vi "Register Broadcast.vi"(0 "CSM Name":string, 1 "TcpRouter-Client in":refnum<class "TcpRouter-Client.lvclass">, 5 "Source CSM Name (* as Default)":string="*", 7 "Status":string, 9 "Response Message (if \"\", same as Source Message)":string, 11 "error in (no error)":errorcluster, 12 "Response Timeout(5000ms)":i32=5000, 13 "Priority (No Change)":T1) -> (4 "CSM Name(dup)":string, 15 "error out":errorcluster)   [LabVIEW 2020, in "CSM-TCP-Router.lvlib" / "TcpRouter-Client.lvclass"]
uses:
  TcpRouter-Client.lvclass
  TcpRouter-Client.lvclass/TcpRouter-Client.ctl
  CSM-TCP-Router.lvlib
  _support/tcp-msg type.ctl
  <userlib>/_NEVSTOP/Communicable State Machine(CSM)/Communicable State Machine.lvlib
  f32241c3-0036-4787-bc41-e9c1f987f5e1.vi
  <userlib>/_NEVSTOP/Communicable State Machine(CSM)/_Polymophic/Build Register Message.vi
  <userlib>/_NEVSTOP/Communicable State Machine(CSM)/AdvanceAPI/CSM - Broadcast Message Type.ctl
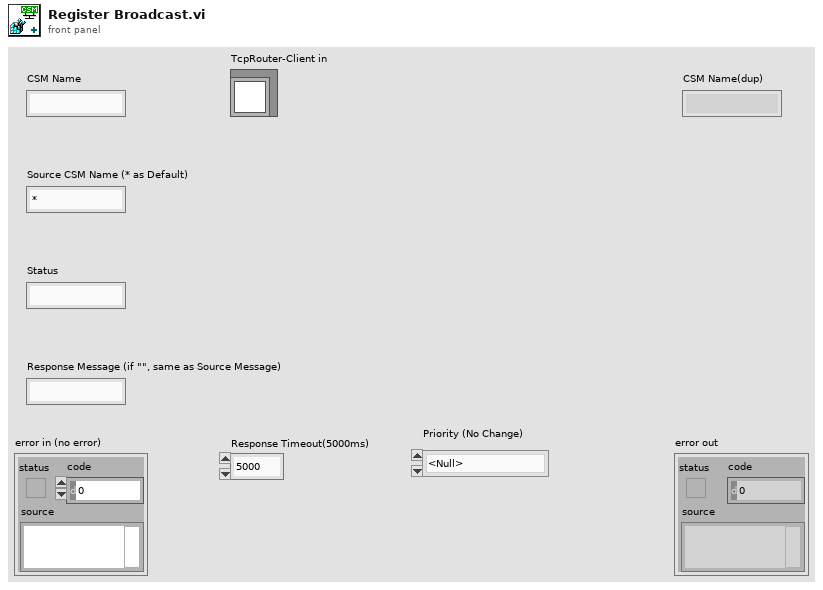
[diagram p1: front panel]
types:
  T1 = typedef "Communicable State Machine.lvlib/CSM - Broadcast Message Type.ctl" = enum16{"<Null>", "Status", "Interrupt"}
  T2 = typedef "CSM-TCP-Router.lvlib/tcp-msg type.ctl" = enum8{"info", "error", "cmd", "cmd-resp", "resp", "async-resp", "status", "interrupt"}
  T3 = typedef "CSM-TCP-Router.lvlib/TcpRouter-Client.lvclass/Def-TCP-Router REQ-REP.ctl" = cluster{"REQ-REP":refnum<k5>}
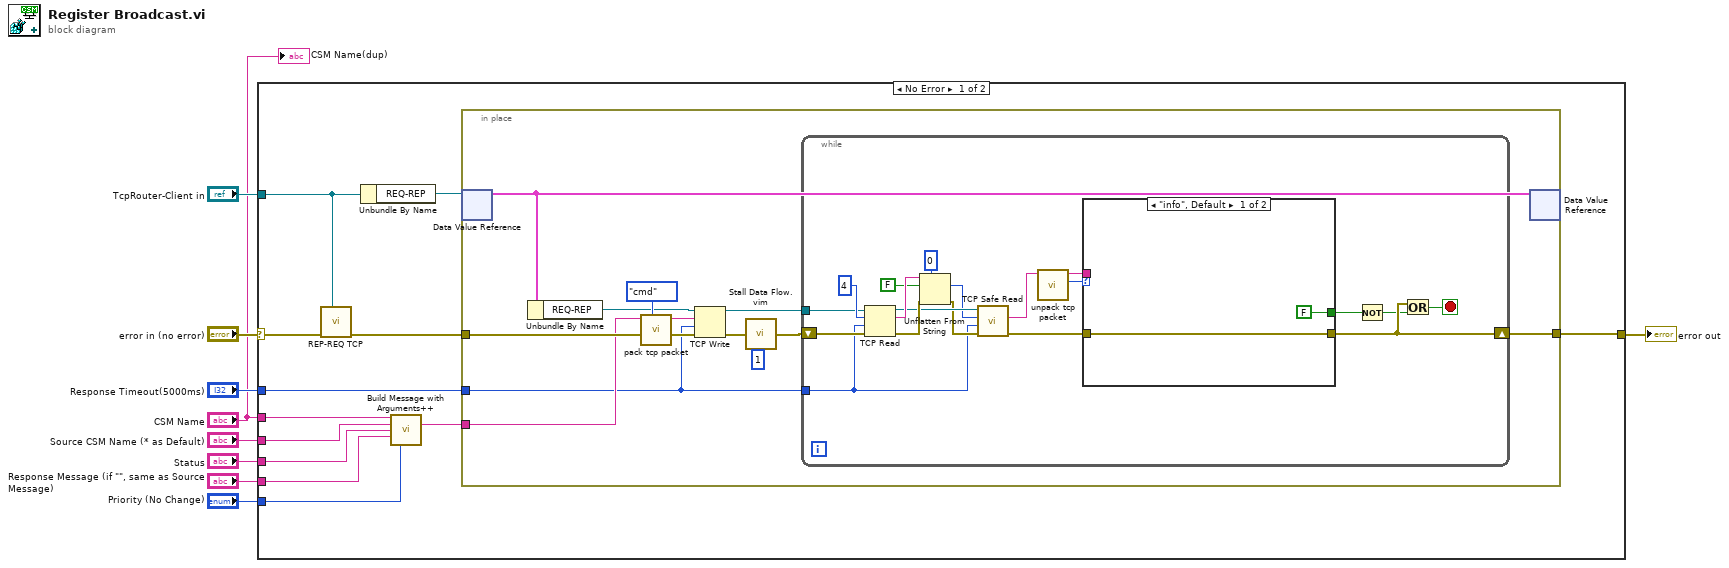
[diagram p0: block diagram]
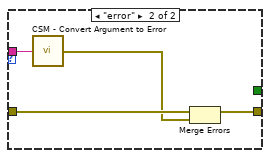
[diagram p2: hidden frame]
diagram:
  n1 = case shown="No Error" "error in (no error)" {
    selector: "error in (no error)" -> [w21 w59]
    tunnel: [w18 w59] -> w8
    tunnel: "TcpRouter-Client in" -> [w16 _]
    tunnel: "Response Timeout(5000ms)" -> [w17 _]
    tunnel: "CSM Name" -> [w13 _]
    tunnel: "Source CSM Name (* as Default)" -> [w14 _]
    tunnel: "Status" -> [w11 _]
    tunnel: "Response Message (if \"\", same as Source Message)" -> [w12 _]
    tunnel: "Priority (No Change)" -> [w10 _]
    frame No Error {
      n2 = call "REP-REQ TCP.vi"("TcpRouter-Client in"=w16, "error in (no error)"=w21) -> ("error out"=w20:errorcluster)  [unwired: 7 in, 2 out]
      n3 = Unbundle By Name(w16) -> ("REQ-REP"=w15:refnum<data-value>)
      n4 = call-poly <userlib>:"Build Message with Arguments++.vi"("Target CSM"=w13, "Source CSM (* as Default)"=w14, "Status"=w11, "API (If \"\", Same As \"Status\")"=w12, "Priority (No Change)"=w10) -> ("CSM Message String"=w19:string)  [unwired: 10 in]
      n5 = in-place {
        in-place-border: w20 -> [w31]
        in-place-border: w19 -> [w30]
        in-place-border: [w25] -> w18
        in-place-border: w17 -> [w24]
        n6 = in-place-dvr #1(w15) -> (w23:T3)  [unwired: 1 out]
        n7 = Unbundle By Name(w23) -> ("REQ-REP"=w22:refnum<k5>)
        n8 = call "pack tcp packet.vi"("tcp-message-type"=tcp-msg_type."cmd", "String"=w30) -> ("TCP Pack"=w33:string)  [unwired: 9 in]
        n9 = TCP Write(connection ID=w22, data in=w33, error in (no error)=w31, 9:w24) -> (connection ID out=w27:refnum<k5>, error out=w29:errorcluster)  [unwired: 1 out]
        n10 = call "Stall Data Flow.vim"("value in"=w29, "milliseconds to wait"=u32 1) -> ("value out"=w26:errorcluster)  [unwired: 1 out]
        n11 = while {
          tunnel: w27 -> [w43]
          shift-right: [w38] -> w25
          shift-left: w26 -> [w42]
          tunnel: w24 -> [w37]
          stop <- w36 stop-if-true
          n12 = TCP Read(connection ID=w43, bytes to read=4, error in (no error)=w42, 9:w37) -> (connection ID out=w50:refnum<k5>, data out=w51:string, error out=w52:errorcluster)  [unwired: 1 in]
          n13 = Unflatten From String(type=0, binary string=w51, data includes array or string size? (T)=FALSE, error in (no error)=w52) -> (value=w48:i32, error out=w47:errorcluster)  [unwired: 2 out]
          n14 = call "TCP Safe Read.vi"("error in (no error)"=w47, "timeout ms (25000)"=w37, "bytes to read"=w48, "TCP Network Connection in"=w50) -> ("error out"=w40:errorcluster, "String"=w49:string)  [unwired: 5 in, 1 out]
          n15 = call "unpack tcp packet.vi"("TCP Pack"=w49) -> ("tcp-message-type"=w41:T2, "String"=w39:string)  [unwired: 9 in]
          n16 = case shown="\"info\", Default" w41 {
            tunnel: w40 -> [w54 w58]
            tunnel: [w54 w56] -> w38
            tunnel: w39 -> [_ w57]
            tunnel: [FALSE _] -> w35
            frame "info", Default {
            }
            frame "error" {
              n17 = call <userlib>:"CSM - Convert Argument to Error.vi"("Argument"=w57) -> ("Error"=w55:errorcluster)  [unwired: 4 in]
              n18 = Merge Errors(w58, w55) -> (w56:errorcluster)
            }
          }
          n19 = Not(x=w35) -> (.not. x?=w34:bool)
          n20 = Or(x=w38, y=w34) -> (x .or. y?=w36:bool)
        }
        n21 = in-place-dvr #1(w23) -> ()  [unwired: 2 out]
      }
    }
    frame Error {
    }
  }
  "error out" <- w8
  "CSM Name(dup)" <- "CSM Name"
